vi "Digital Pin Mode.vi"() -> ()   [LabVIEW 2011, in "LVH-LINX.lvlib"]
uses:
  LVH-LINX.lvlib
panel:
  in  "Digital Pin Mode":enum16{"Input", "Output"}(ring)
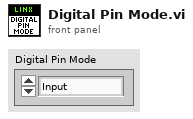
[diagram p1: front panel]
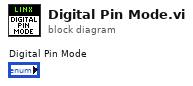
[diagram p0: block diagram]
diagram:
